vi "SetupGlobals.vi"() -> ()   [LabVIEW 2019]
uses:
  Sub Controls/Instrument IDN.ctl
panel:
  in  "Instrument List":T1[](array[typedef]) {"Status" format="%.0x"}
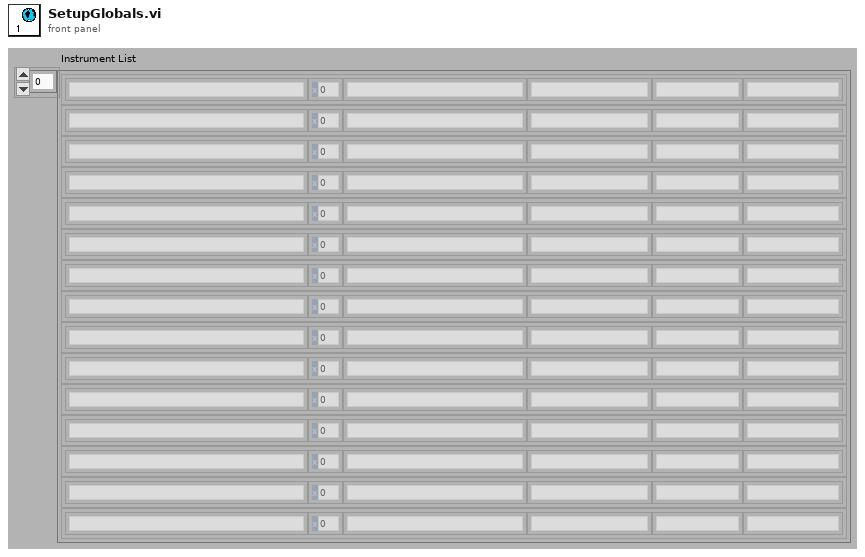
[diagram p1: front panel]
types:
  T1 = typedef "Instrument IDN.ctl" = cluster{"VISA Address":string, "Status":u16, "Manufacturer":string, "Model":string, "Info":string, "Info 2":string, "Misc Data":variant}
diagram:
